vi "Load LCOS Correction Pattern.vi"(0 "Images Dest":T1, 3 "error in":errorcluster) -> (5 "Cancelled?":bool, 6 "Images Out":T1, 7 "Correct File Type":bool, 8 "Path":path, 9 "error out":errorcluster)   [LabVIEW 2011]
uses:
  LCOS Images.ctl
  <vilib>/vision/Image Controls.llb/IMAQ Image.ctl
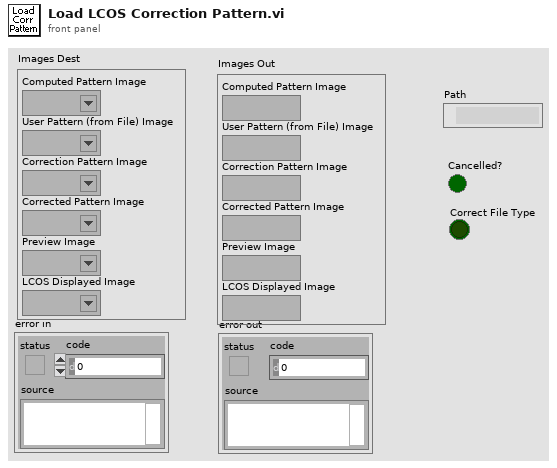
[diagram p1: front panel]
types:
  T1 = typedef "LCOS Images.ctl" = cluster{"Computed Pattern Image":T2, "User Pattern (from File) Image":T2, "Correction Pattern Image":T2, "Corrected Pattern Image":T2, "Preview Image":T2, "LCOS Displayed Image":T2}
  T2 = typedef "IMAQ Image.ctl" = refnum<image>
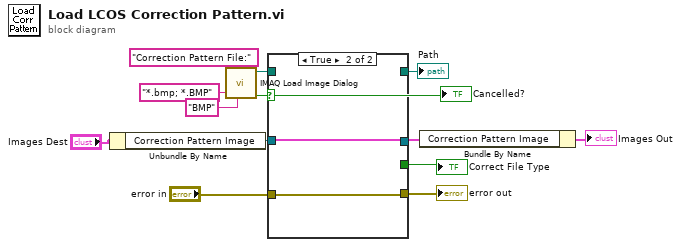
[diagram p0: block diagram]
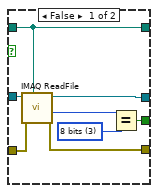
[diagram p2: hidden frame]
diagram:
  n1 = Unbundle By Name("Images Dest") -> ("Correction Pattern Image"=w5:T2)
  n2 = call "IMAQ Load Image Dialog"("Pattern Label"="BMP", "Prompt"="Correction Pattern File:", "Pattern"="*.bmp; *.BMP") -> ("Cancelled?"=w7:bool, "Path"=w6:path)  [unwired: 6 in, 1 out]
  "Cancelled?" <- w7
  n3 = case shown="True" w7 {
    tunnel: w5 -> [w15 w23]
    tunnel: [w21 w23] -> w2
    tunnel: "error in" -> [w20 w22]
    tunnel: [w19 w22] -> w12
    tunnel: [w17 _] -> w11
    tunnel: w6 -> [w14 _]
    tunnel: [w14 _] -> w1
    frame False {
      w16 = 3 items=["1 bit", "2 bits", "4 bits", "8 bits", "12 bits (unsigned)", "16 bits (unsigned)", "16 bits (signed)", "16 bits (RGB chunky)", "24 bits (RGB chunky)", "24 bits (RGB planar)", "32 bits (unsigned)", "32 bits (signed)", "32 bits (RGB chunky)", "32 bits (float)", "48 bits (Complex 2x24 int)", "64 bits (Complex 2x32 float)", "reserved", "24 bits (HSL)", "48 bits (RGB chunky)", "64 bits (RGB chunky)"] ("File Data Type")
      n4 = call "IMAQ ReadFile"("File Path"=w14, "error in (no error)"=w20, "Image"=w15) -> ("error out"=w19:errorcluster, "File Data Type out"=w18:i32, "Image Out"=w21:T2)  [unwired: 4 in, 2 out]
      n5 = Equal?(x=w18, y=w16) -> (x = y?=w17:bool)
    }
    frame True {
    }
  }
  "error out" <- w12
  "Correct File Type" <- w11
  "Path" <- w1
  n6 = Bundle By Name(cluster="Images Dest", "Correction Pattern Image"=w2) -> (→"Images Out":T1)
